vi "Word Example.vi"() -> ()   [LabVIEW 2017]
doc: "This example shows how to use the LabVIEW NPOI library to manipulate MS Word Files."
uses:
  LabVIEW NPOI/MS-Word/MS-Word.lvclass
  C:/Users/Neo/Desktop/Dev_Tools_BR/LabVIEW_NPOI/src/LabVIEW NPOI/Document/Document.lvclass
  <vilib>/Utility/sysdir.llb/System Directory Type.ctl
  LabVIEW NPOI/Document/Document.lvclass/Document.ctl
  LabVIEW NPOI/Document/Get FilePath.vi
  082b00c0-f2da-4da4-bdc9-d000497b5f47.vi
  LabVIEW NPOI/Document/Read Table As String.vi
  LabVIEW NPOI/Document/Append Table (string).vi
  LabVIEW NPOI/Document/Append Table (double).vi
  LabVIEW NPOI/Document/Document.lvclass
panel:
  in  "print":bool
  in  "createDocumentBttn":bool
  in  "Text":string="Lorem ipsum dolor sit amet, consectetur adipiscing elit, sed do eiusmod tempor incididunt ut labore et dolore magna aliqua. Adipiscing bibendum est ultricies integer quis auctor elit sed vulputate. Volutpat consequat mauris nunc congue nisi vitae suscipit tellus. Eget arcu dictum varius duis at consectetur lorem donec massa. Morbi enim nunc faucibus a pellentesque sit. Risus ultricies tristique nulla aliquet enim tortor at. Sit amet consectetur adipiscing elit ut aliquam purus sit. Porta lorem mollis aliquam ut porttitor leo a diam. Odio aenean sed adipiscing diam donec adipiscing tristique risus. Nunc eget lorem dolor sed viverra ipsum nunc aliquet. Ultrices gravida dictum fusce ut. Mi eget mauris pharetra et ultrices. Ultrices dui sapien eget mi proin. Duis ut diam quam nulla porttitor massa id neque. Eu lobortis elementum nibh tellus molestie nunc non. Iaculis nunc sed augue lacus viverra. Enim sed faucibus turpis in eu. Quis viverra nibh cras pulvinar mattis. Auctor augue mauris augue neque gravida. Enim ut tellus elementum sagittis vitae."
  in  "addParagraphBttn":bool
  in  "HTML File Path":path
  in  "convertToHtml":bool
  out "Read Table Time":u32
  out "Add Table Time":u32
  in  "addImageBttn":bool
  out "Table Control":string[][](table)
  in  "readTableBttn":bool
  in  "#Columns":i32=100
  in  "#Rows":i32=2
  in  "tableType":enum32{"Strings", "Doubles"}(radio)
  in  "addTableBttn":bool
  out "FilePath":path
  in  "openDocumentBttn":bool
  in  "baseDocumentPath":path caption="Folder Path"
  in  "saveAsDocumentBttn":bool
  in  "saveDocumentBttn":bool
  in  "documentName":string="Book1.xlsx" caption="Name"
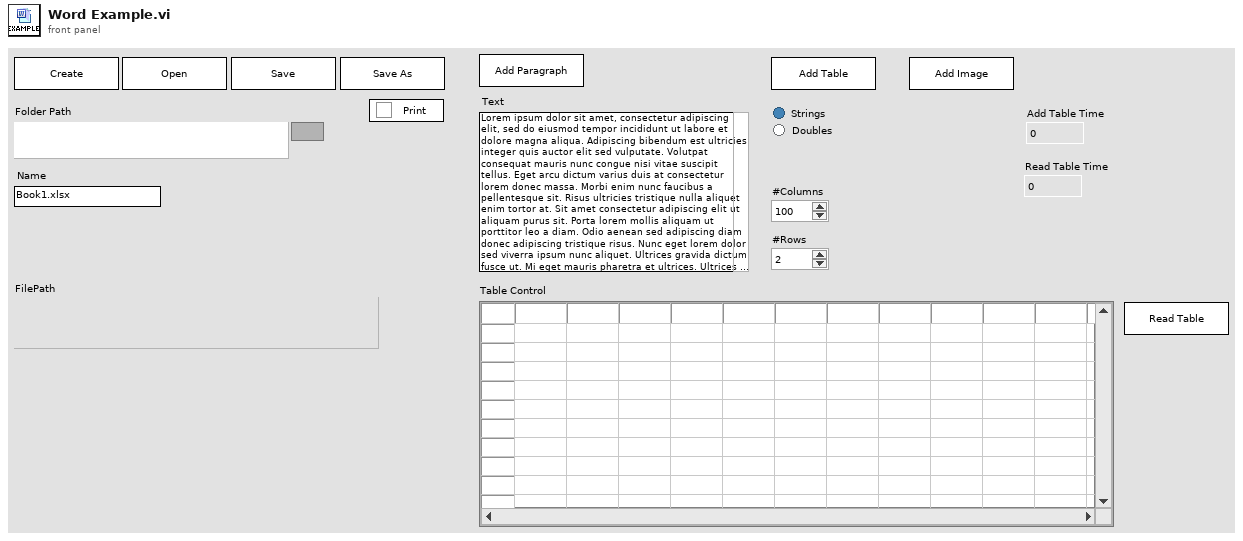
[diagram p1: front panel]
types:
  T1 = typedef "System Directory Type.ctl" = i32
  T2 = cluster{"documentObject":refnum<class "MS-Word.lvclass">, "documentPath":path, "documentName":string, "pageName":string, "styleName":string, "ctlRefs":refnum<vi>[]}
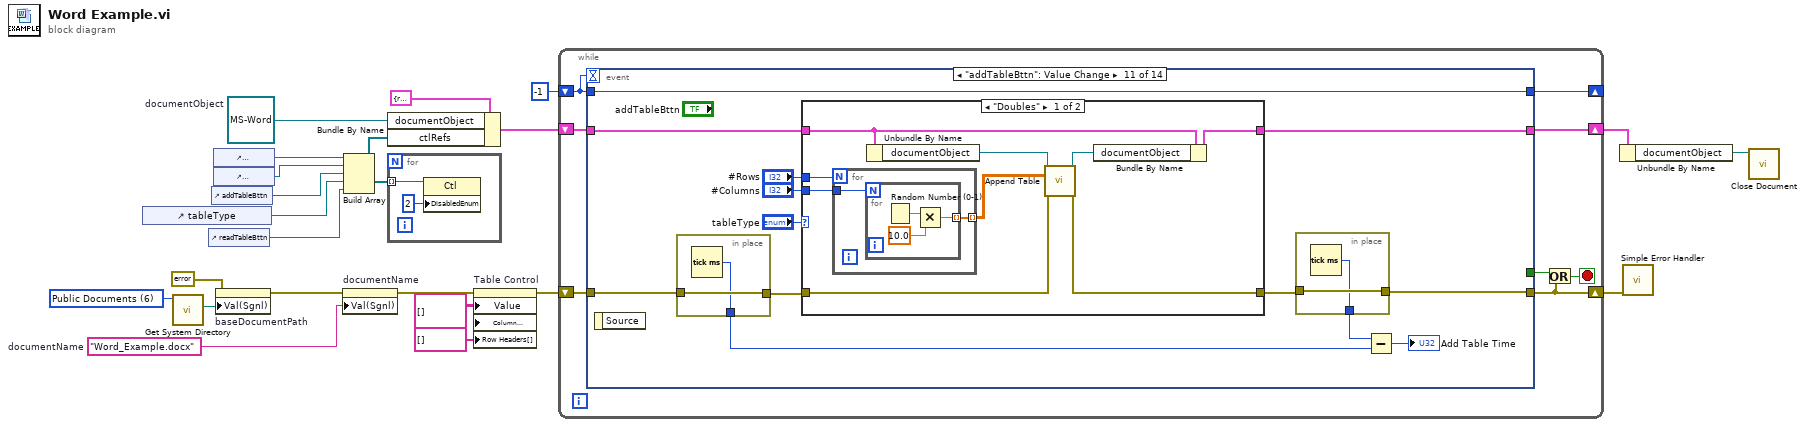
[diagram p0: block diagram]
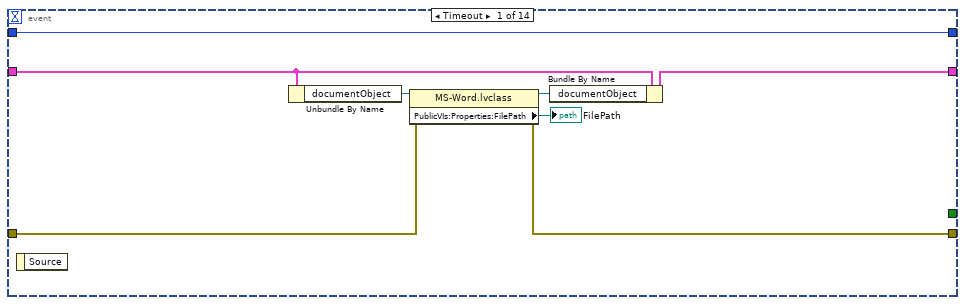
[diagram p2: hidden frame]
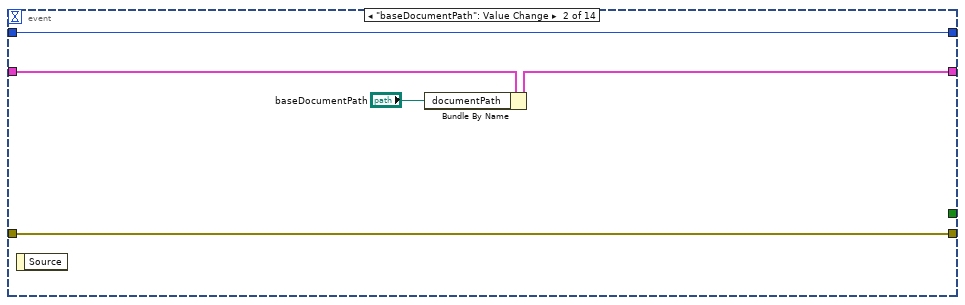
[diagram p3: hidden frame]
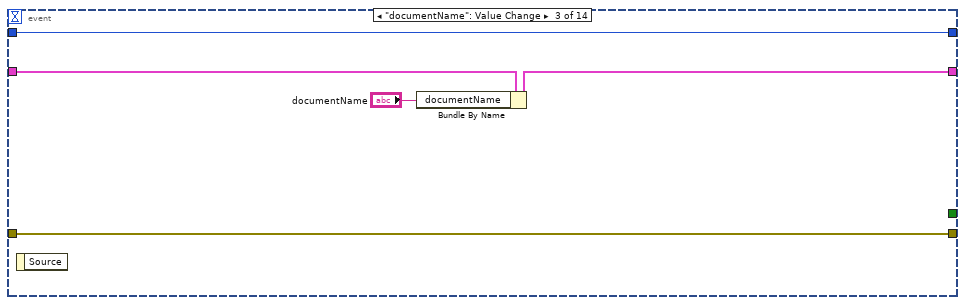
[diagram p4: hidden frame]
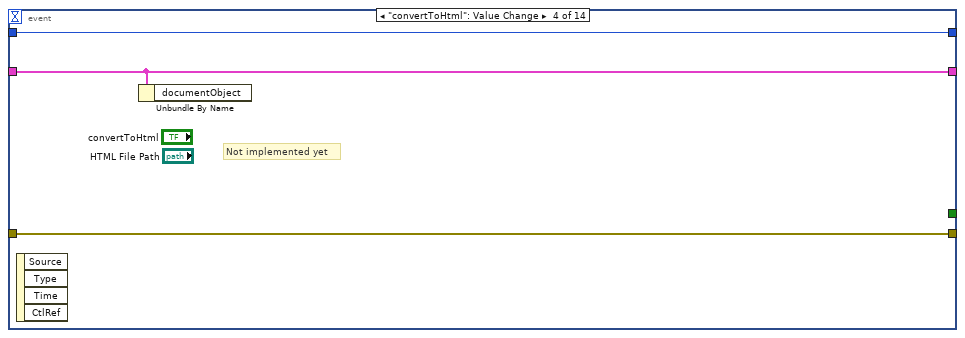
[diagram p5: hidden frame]
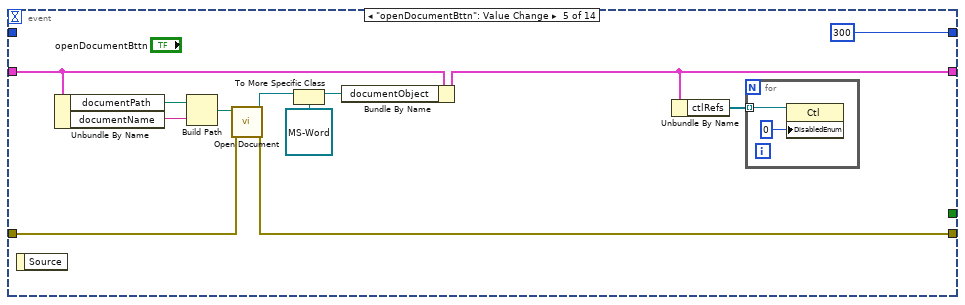
[diagram p6: hidden frame]
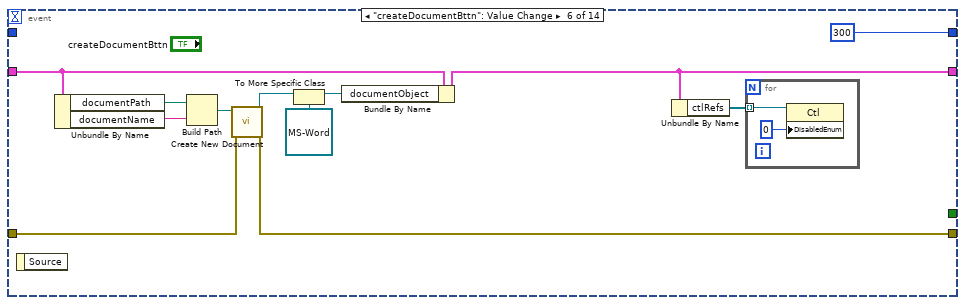
[diagram p7: hidden frame]
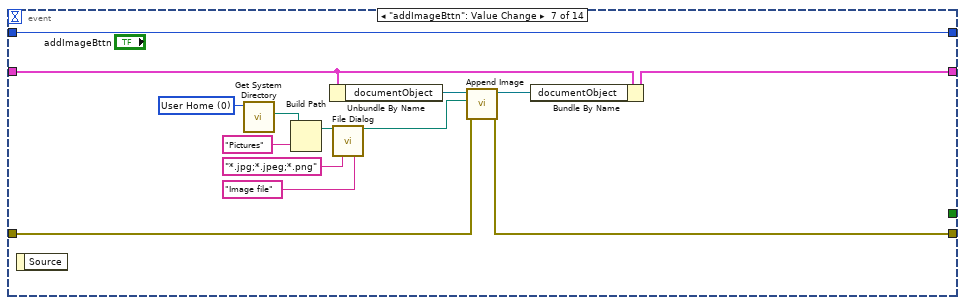
[diagram p8: hidden frame]
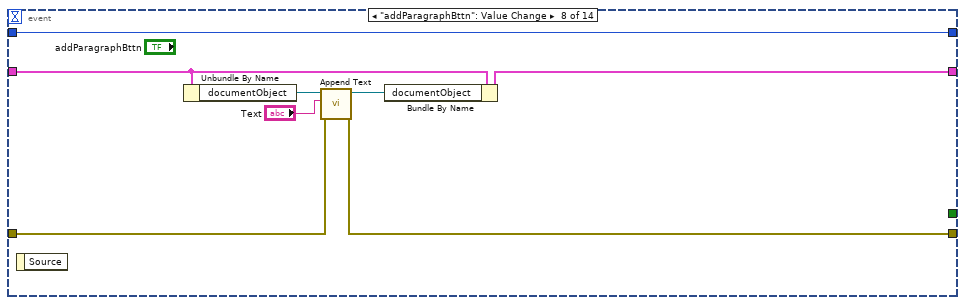
[diagram p9: hidden frame]
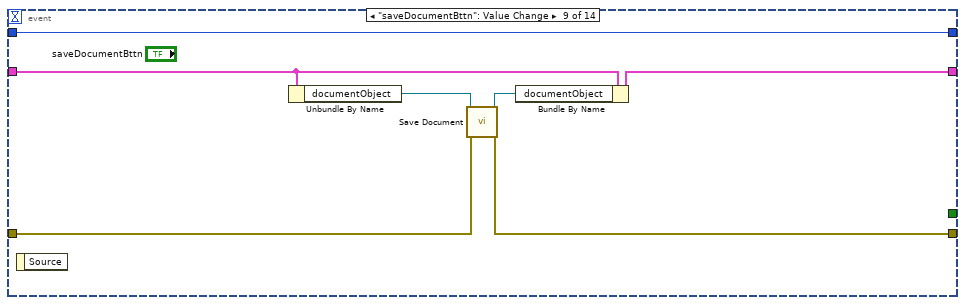
[diagram p10: hidden frame]
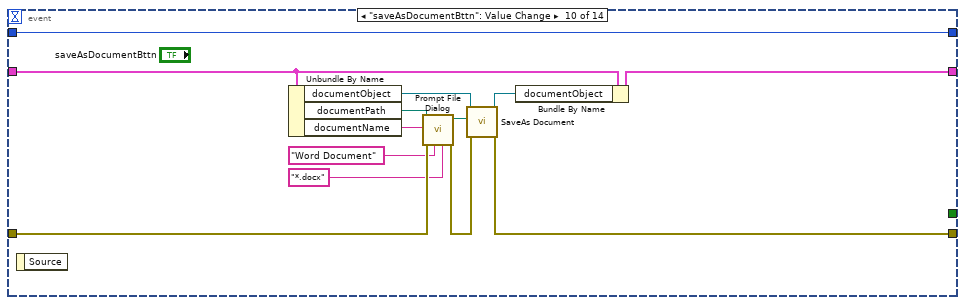
[diagram p11: hidden frame]
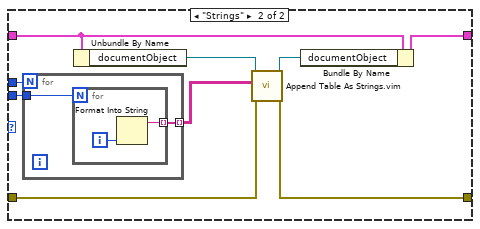
[diagram p12: hidden frame]
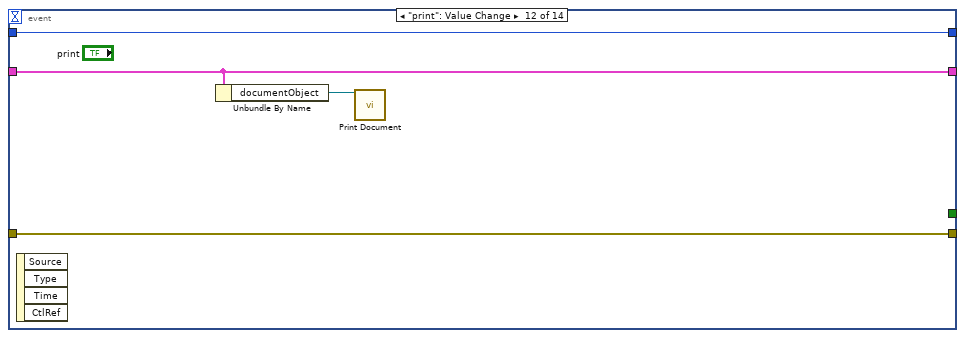
[diagram p13: hidden frame]
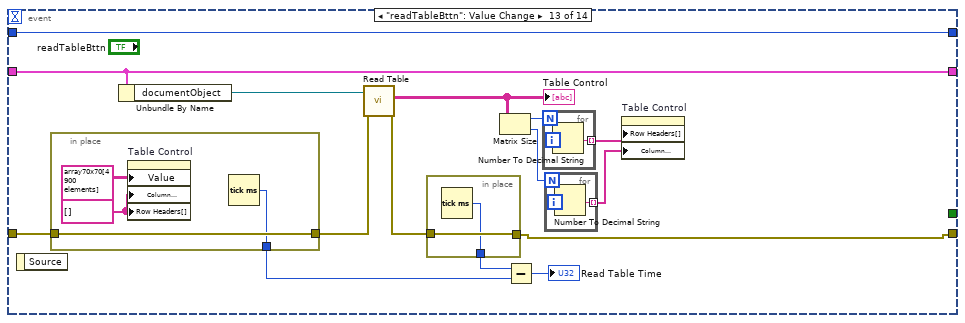
[diagram p14: hidden frame]
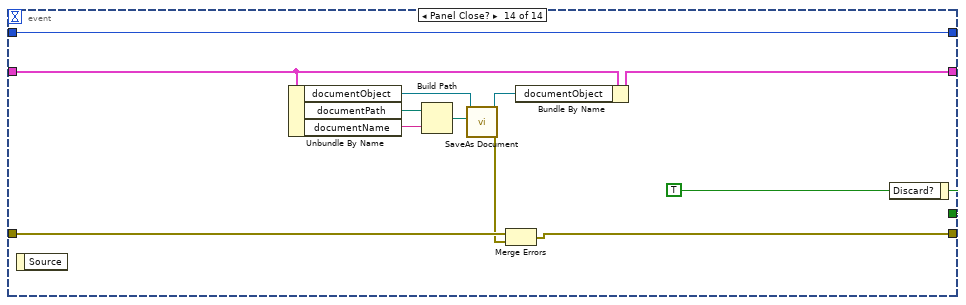
[diagram p15: hidden frame]
diagram:
  w2 = T1 6 items=["User Home"=0, "User Desktop"=1, "User Documents"=2, "User Application Data"=3, "User Preferences"=4, "User Temporary"=5, "Public Documents"=6, "Public Application Data"=7, "Public Preferences"=8, "Public Cache"=13, "System Core Libraries"=9, "System Installed Libraries"=10, "Application Files"=11, "Boot Volume Root"=12] ("system directory type")
  w7 = string[] [] ("Row Header Strings[]")
  w12 = "Word_Example.docx"  # documentName
  w16 = refnum<class "MS-Word.lvclass"> refnum  # documentObject
  n1 = control-ref of="tableType"() -> (w10:refnum<vi>)
  n2 = call <vilib>:"Get System Directory.vi"("system directory type"=w2) -> ("system directory"=w1:path)  [unwired: 10 in]
  n3 = control-ref of="readTableBttn"() -> (w9:refnum<vi>)
  n4 = control-ref of="addTableBttn"() -> (w11:refnum<vi>)
  n5 = control-ref of="saveDocumentBttn"() -> (w15:refnum<vi>)
  n6 = control-ref of="saveAsDocumentBttn"() -> (w14:refnum<vi>)
  n7 = property on="baseDocumentPath" class="Path"(error in=errorcluster {"status"=FALSE, "code"=0, "source"=""} ("error IO"), "Val(Sgnl)"=w1) -> (error out=w6:errorcluster)  [unwired: 1 in, 1 out]
  n8 = property on="documentName" class="Str"(error in=w6, "Val(Sgnl)"=w12) -> (error out=w5:errorcluster)  [unwired: 1 in, 1 out]
  n9 = Build Array(w15, w14, w11, w10, w9) -> (w13:refnum<vi>[])
  n10 = Bundle By Name(cluster=T2 {"documentObject"=refnum, "documentPath"=path "", "documentName"="", "pageName"="", "styleName"="Default", "ctlRefs"=[]}, "documentObject"=w16, "ctlRefs"=w13) -> (w22:T2)
  n11 = for {
    tunnel: w13 -> [w24] mode=indexing
    n12 = property class="Ctl"(reference=w24, "DisabledEnum"=u8 2) -> ()  [unwired: 1 in, 2 out]
  }
  n13 = property on="Table Control" class="Tbl (strict)"(error in=w5, "Value"=string[][] [] ("Table Control"), "Column Headers[]"=w7, "Row Headers[]"=w7) -> (error out=w3:errorcluster)  [unwired: 1 in, 1 out]
  n14 = while {
    shift-right: [w31] -> w19
    shift-left: w22 -> [w32]
    shift-right: [w29] -> w21
    shift-left: w3 -> [w30]
    shift-right: [w25] -> _
    shift-left: -1 -> [w26]
    stop <- w27 stop-if-true
    n15 = event shown="[10] \"addTableBttn\": Value Change" {
      selector: _ -> [_ _ _ _ _ _ _ _ _ _ _ _ _ _]
      dyn-events: _ -> [_ _ _ _ _ _ _ _ _ _ _ _ _ _]
      timeout: w26 -> [_ _ _ _ _ _ _ _ _ _ _ _ _ _]
      tunnel: [_ _ _ _ _ _ _ _ _ _ _ _ _ w201] -> w28
      tunnel: w32 -> [w40 w45 w50 w51 w65 w79 w94 w102 w110 w123 w131 w169 w185 w208]
      tunnel: [w33 w44 w49 w51 w60 w74 w90 w98 w108 w121 w136 w169 w185 w203] -> w31
      tunnel: [w36 w42 w47 w53 w54 w68 w91 w99 w106 w119 w127 w171 w175 w199] -> w29
      tunnel: w30 -> [w37 w42 w47 w53 w62 w76 w92 w100 w105 w117 w130 w171 w178 w200]
      tunnel: w26 -> [w34 w41 w46 w52 _ _ w95 w103 w104 w111 w135 w170 w186 w197]
      tunnel: [w34 w41 w46 w52 300 300 w95 w103 w104 w111 w135 w170 w186 w197] -> w25
      event Timeout {
        n16 = event-data() -> ()  [unwired: 1 in, 1 out]
        n17 = Unbundle By Name(w40) -> ("documentObject"=w39:refnum<class "MS-Word.lvclass">)
        n18 = property class="MS-Word.lvclass"(reference=w39, error in=w37) -> (reference out=w38:refnum<class "MS-Word.lvclass">, error out=w36:errorcluster, "PublicVIs:Properties:FilePath"=→"FilePath":path)
        n19 = Bundle By Name(cluster=w40, "documentObject"=w38) -> (w33:T2)
      }
      event "baseDocumentPath": Value Change {
        n20 = event-data() -> ()  [unwired: 1 in, 1 out]
        n21 = Bundle By Name(cluster=w45, "documentPath"="baseDocumentPath") -> (w44:T2)
      }
      event "documentName": Value Change {
        n22 = event-data() -> ()  [unwired: 1 in, 1 out]
        n23 = Bundle By Name(cluster=w50, "documentName"="documentName") -> (w49:T2)
      }
      event "convertToHtml": Value Change {
        # "Not implemented yet"
        n24 = event-data() -> ()  [unwired: 1 in, 4 out]
        n25 = Unbundle By Name(w51) -> ()  [unwired: 1 out]
      }
      event "openDocumentBttn": Value Change {
        n26 = event-data() -> ()  [unwired: 1 in, 1 out]
        n27 = Unbundle By Name(w65) -> ("documentPath"=w64:path, "documentName"=w63:string)
        n28 = Build Path(base path=w64, name or relative path=w63) -> (appended path=w58:path)
        n29 = call "Open Document.vi"("error in (no error)"=w62, "File Path"=w58) -> ("error out"=w54:errorcluster, "Document out"=w56:refnum<class "Document.lvclass">)  [unwired: 8 in]
        n30 = To More Specific Class(target class=refnum<class "MS-Word.lvclass"> refnum ("workbookObject"), reference=w56) -> (specific class reference=w55:refnum<class "MS-Word.lvclass">)  [unwired: 1 in, 1 out]
        n31 = Bundle By Name(cluster=w65, "documentObject"=w55) -> (w60:T2)
        n32 = Unbundle By Name(w60) -> ("ctlRefs"=w59:refnum<vi>[])
        n33 = for {
          tunnel: w59 -> [w67] mode=indexing
          n34 = property class="Ctl"(reference=w67, "DisabledEnum"=u8 0) -> ()  [unwired: 1 in, 2 out]
        }
      }
      event "createDocumentBttn": Value Change {
        n35 = event-data() -> ()  [unwired: 1 in, 1 out]
        n36 = Unbundle By Name(w79) -> ("documentPath"=w78:path, "documentName"=w77:string)
        n37 = Build Path(base path=w78, name or relative path=w77) -> (appended path=w72:path)
        n38 = call "Create New Document.vi"("error in (no error)"=w76, "File Path"=w72) -> ("error out"=w68:errorcluster, "Document out"=w70:refnum<class "Document.lvclass">)  [unwired: 8 in]
        n39 = To More Specific Class(target class=refnum<class "MS-Word.lvclass"> refnum ("workbookObject"), reference=w70) -> (specific class reference=w69:refnum<class "MS-Word.lvclass">)  [unwired: 1 in, 1 out]
        n40 = Bundle By Name(cluster=w79, "documentObject"=w69) -> (w74:T2)
        n41 = Unbundle By Name(w74) -> ("ctlRefs"=w73:refnum<vi>[])
        n42 = for {
          tunnel: w73 -> [w81] mode=indexing
          n43 = property class="Ctl"(reference=w81, "DisabledEnum"=u8 0) -> ()  [unwired: 1 in, 2 out]
        }
      }
      event "addImageBttn": Value Change {
        w84 = T1 0 items=["User Home"=0, "User Desktop"=1, "User Documents"=2, "User Application Data"=3, "User Preferences"=4, "User Temporary"=5, "Public Documents"=6, "Public Application Data"=7, "Public Preferences"=8, "Public Cache"=13, "System Core Libraries"=9, "System Installed Libraries"=10, "Application Files"=11, "Boot Volume Root"=12] ("system directory type")
        n44 = event-data() -> ()  [unwired: 1 in, 1 out]
        n45 = call <vilib>:"Get System Directory.vi"("system directory type"=w84) -> ("system directory"=w85:path)  [unwired: 10 in]
        n46 = Build Path(base path=w85, name or relative path="Pictures") -> (appended path=w83:path)
        n47 = Unbundle By Name(w94) -> ("documentObject"=w93:refnum<class "MS-Word.lvclass">)
        n48 = call "File Dialog"("start path"=w83, "pattern (all files)"="*.jpg;*.jpeg;*.png", "pattern label"="Image file") -> ("selected path"=w88:path)  [unwired: 9 in, 3 out]
        n49 = call "Append Image.vi"("error in (no error)"=w92, "Image File Path"=w88, "Document in"=w93) -> ("error out"=w91:errorcluster, "Document out"=w89:refnum<class "MS-Word.lvclass">)  [unwired: 7 in]
        n50 = Bundle By Name(cluster=w94, "documentObject"=w89) -> (w90:T2)
      }
      event "addParagraphBttn": Value Change {
        n51 = event-data() -> ()  [unwired: 1 in, 1 out]
        n52 = Unbundle By Name(w102) -> ("documentObject"=w101:refnum<class "MS-Word.lvclass">)
        n53 = call "Append Text.vi"("error in (no error)"=w100, "Text"="Text", "Document in"=w101) -> ("error out"=w99:errorcluster, "Document out"=w97:refnum<class "MS-Word.lvclass">)  [unwired: 7 in]
        n54 = Bundle By Name(cluster=w102, "documentObject"=w97) -> (w98:T2)
      }
      event "saveDocumentBttn": Value Change {
        n55 = event-data() -> ()  [unwired: 1 in, 1 out]
        n56 = Unbundle By Name(w110) -> ("documentObject"=w109:refnum<class "MS-Word.lvclass">)
        n57 = call "Save Document.vi"("error in (no error)"=w105, "Document in"=w109) -> ("error out"=w106:errorcluster, "Document out"=w107:refnum<class "MS-Word.lvclass">)  [unwired: 8 in]
        n58 = Bundle By Name(cluster=w110, "documentObject"=w107) -> (w108:T2)
      }
      event "saveAsDocumentBttn": Value Change {
        n59 = event-data() -> ()  [unwired: 1 in, 1 out]
        n60 = Unbundle By Name(w123) -> ("documentObject"=w122:refnum<class "MS-Word.lvclass">, "documentPath"=w113:path, "documentName"=w112:string)
        n61 = call "Prompt File Dialog.vi"("pattern (all files)"="*.docx", "pattern label"="Word Document", "error in"=w117, "default name"=w112, "File Path"=w113) -> ("error out"=w116:errorcluster, "selected path"=w118:path)  [unwired: 5 in]
        n62 = call "SaveAs Document.vi"("error in (no error)"=w116, "File Path"=w118, "Document in"=w122) -> ("error out"=w119:errorcluster, "Document out"=w120:refnum<class "MS-Word.lvclass">)  [unwired: 7 in]
        n63 = Bundle By Name(cluster=w123, "documentObject"=w120) -> (w121:T2)
      }
      event "addTableBttn": Value Change {
        n64 = event-data() -> ()  [unwired: 1 in, 1 out]
        n65 = in-place {
          in-place-border: w130 -> [w140]
          in-place-border: [w140] -> w129
          in-place-border: [w139] -> w125
          n66 = Tick Count (ms)() -> (millisecond timer value=w139:u32)
        }
        n67 = case shown="\"Doubles\"" "tableType" {
          tunnel: w131 -> [w149 w163]
          tunnel: [w147 w161] -> w136
          tunnel: [w145 w159] -> w128
          tunnel: w129 -> [w144 w158]
          tunnel: "#Columns" -> [w141 w156]
          tunnel: "#Rows" -> [w142 w155]
          frame "Doubles" {
            n68 = for {
              N: w142 -> [_]
              tunnel: [w151] -> w143 mode=indexing
              tunnel: w141 -> [w150]
              n69 = for {
                N: w150 -> [_]
                tunnel: [w153] -> w151 mode=indexing
                n70 = Random Number (0-1)() -> (number: 0 to 1=w154:dbl)
                n71 = Multiply(x=w154, y=10.0) -> (x*y=w153:dbl)
              }
            }
            n72 = Unbundle By Name(w149) -> ("documentObject"=w148:refnum<class "MS-Word.lvclass">)
            n73 = call-poly "Append Table.vi"("Document in"=w148, "Table"=w143, "error in (no error)"=w144) -> ("Document out"=w146:refnum<class "MS-Word.lvclass">, "error out"=w145:errorcluster)  [unwired: 11 in]
            n74 = Bundle By Name(cluster=w149, "documentObject"=w146) -> (w147:T2)
          }
          frame "Strings" {
            n75 = for {
              N: w155 -> [_]
              tunnel: [w165] -> w157 mode=indexing
              tunnel: w156 -> [w164]
              n76 = for {
                N: w164 -> [_]
                tunnel: [w166] -> w165 mode=indexing
                i -> [w167]
                n77 = Format Into String(w167) -> (resulting string=w166:string)  [unwired: 3 in, 1 out]
              }
            }
            n78 = Unbundle By Name(w163) -> ("documentObject"=w162:refnum<class "MS-Word.lvclass">)
            n79 = call "Append Table As Strings.vim"("error in (no error)"=w158, "Table"=w157, "Document in"=w162) -> ("error out"=w159:errorcluster, "Document out"=w160:refnum<class "MS-Word.lvclass">)  [unwired: 7 in]
            n80 = Bundle By Name(cluster=w163, "documentObject"=w160) -> (w161:T2)
          }
        }
        n81 = in-place {
          in-place-border: w128 -> [w138]
          in-place-border: [w138] -> w127
          in-place-border: [w137] -> w126
          n82 = Tick Count (ms)() -> (millisecond timer value=w137:u32)
        }
        n83 = Subtract(x=w126, y=w125) -> (x-y=→"Add Table Time":u32)
      }
      event "print": Value Change {
        n84 = event-data() -> ()  [unwired: 1 in, 4 out]
        n85 = Unbundle By Name(w169) -> ("documentObject"=w168:refnum<class "MS-Word.lvclass">)
        n86 = call "Print Document.vi"("Document in"=w168) -> ()  [unwired: 9 in, 2 out]
      }
      event "readTableBttn": Value Change {
        n87 = event-data() -> ()  [unwired: 1 in, 1 out]
        n88 = in-place {
          in-place-border: w178 -> [w190]
          in-place-border: [w190] -> w177
          in-place-border: [w189] -> w173
          w192 = string[] [] ("Row Header Strings[]")
          n89 = property on="Table Control" class="Tbl (strict)"("Value"=string[][] array70x70[4900 elements] ("Table Control"), "Column Headers[]"=w192, "Row Headers[]"=w192) -> ()  [unwired: 2 in, 2 out]
          n90 = Tick Count (ms)() -> (millisecond timer value=w189:u32)
        }
        n91 = Unbundle By Name(w185) -> ("documentObject"=w184:refnum<class "MS-Word.lvclass">)
        n92 = call-poly "Read Table.vi"("error in (no error)"=w177, "Document in"=w184) -> ("error out"=w176:errorcluster, "Table As String"=w183:string[][])  [unwired: 7 in, 1 out]
        "Table Control" <- w183
        n93 = in-place {
          in-place-border: w176 -> [w188]
          in-place-border: [w188] -> w175
          in-place-border: [w187] -> w174
          n94 = Tick Count (ms)() -> (millisecond timer value=w187:u32)
        }
        n95 = Matrix Size(0:w183) -> (1:w182:i32, 2:w180:i32)
        n96 = Subtract(x=w174, y=w173) -> (x-y=→"Read Table Time":u32)
        n97 = for {
          N: w182 -> [_]
          tunnel: [w195] -> w181 mode=indexing
          i -> [w196]
          n98 = Number To Decimal String(number=w196) -> (decimal integer string=w195:string)  [unwired: 1 in]
        }
        n99 = for {
          N: w180 -> [_]
          tunnel: [w193] -> w179 mode=indexing
          i -> [w194]
          n100 = Number To Decimal String(number=w194) -> (decimal integer string=w193:string)  [unwired: 1 in]
        }
        n101 = property on="Table Control" class="Tbl (strict)"("Row Headers[]"=w181, "Column Headers[]"=w179) -> ()  [unwired: 2 in, 2 out]
      }
      event Panel Close? {
        w201 = TRUE ("Discard?")
        n102 = event-data() -> ()  [unwired: 1 in, 1 out]
        n103 = Unbundle By Name(w208) -> ("documentObject"=w205:refnum<class "MS-Word.lvclass">, "documentPath"=w207:path, "documentName"=w206:string)
        n104 = Build Path(base path=w207, name or relative path=w206) -> (appended path=w204:path)
        n105 = call "SaveAs Document.vi"("File Path"=w204, "Document in"=w205) -> ("error out"=w198:errorcluster, "Document out"=w202:refnum<class "MS-Word.lvclass">)  [unwired: 8 in]
        n106 = Merge Errors(w200, w198) -> (w199:errorcluster)
        n107 = Bundle By Name(cluster=w208, "documentObject"=w202) -> (w203:T2)
        n108 = event-data("Discard?"=w201) -> ()  [unwired: 1 in, 1 out]
      }
    }
    n109 = Or(x=w28, y=w29) -> (x .or. y?=w27:bool)
  }
  n110 = Unbundle By Name(w19) -> ("documentObject"=w18:refnum<class "MS-Word.lvclass">)
  n111 = call <vilib>:"Simple Error Handler.vi"("error in (no error)"=w21) -> ()  [unwired: 4 in, 5 out]
  n112 = call "Close Document.vi"("Document in"=w18) -> ()  [unwired: 10 in, 1 out]
